vi "DIO_Configure.vi"(7 "Device Index":i32 format="%.0g", 8 "error in (no error)":errorcluster, 9 "OutBytes":T1 {"Out Byte 3" format="%08b"; "Out Byte 2" format="%08b"; "Out Byte 1" format="%08b"; "Out Byte 0" format="%08b"}, 10 "Out Mask":T2, 11 "Tri State":enum8{"False", "True"}(ring)) -> (0 "error out":errorcluster)   [LabVIEW 2012]
doc: "This VI is used to configure ACCES USB-DIO devices."
uses:
  Controls/DIO_bitMask.ctl
  Controls/DIO_bytemask.ctl
  Windows/System32/AIOUSB.dll
panel:
  out "Return Value":u32 format="%.0g"
  # "Output Bytes"
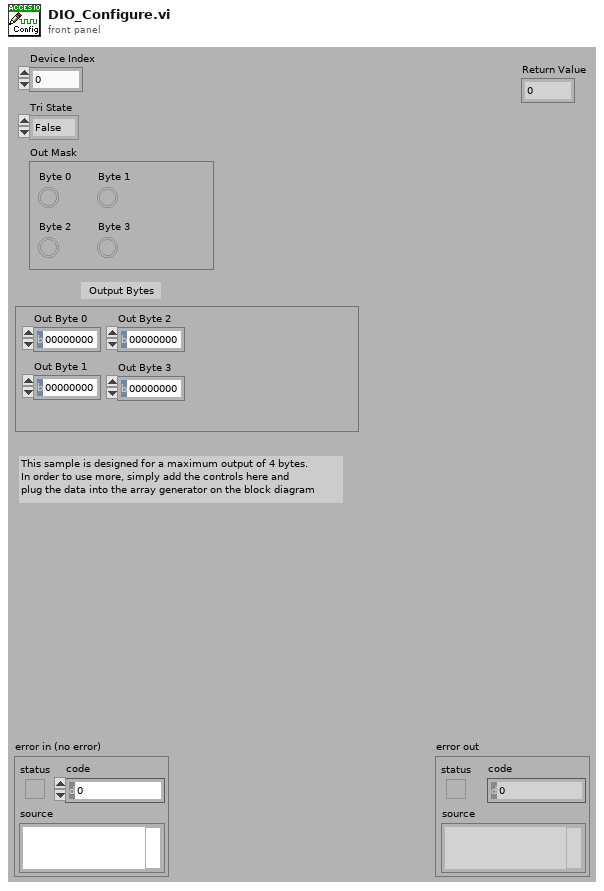
[diagram p1: front panel]
types:
  T1 = typedef "DIO_bytemask.ctl" = cluster{"Out Byte 0":u8, "Out Byte 1":u8, "Out Byte 2":u8, "Out Byte 3":u8}
  T2 = typedef "DIO_bitMask.ctl" = cluster{"Byte 0":bool, "Byte 1":bool, "Byte 2":bool, "Byte 3":bool}
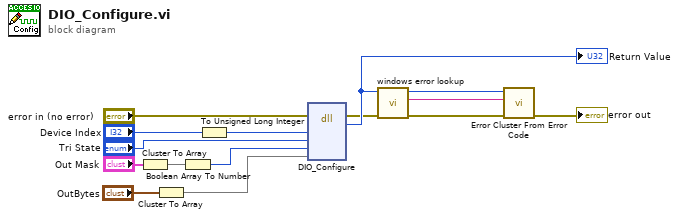
[diagram p0: block diagram]
diagram:
  n1 = Cluster To Array(cluster="Out Mask") -> (array=w3:bool[])
  n2 = Cluster To Array(cluster="OutBytes") -> (array=w5:u8[])
  n3 = Boolean Array To Number(Boolean array=w3) -> (number=w2:u32)
  n4 = To Unsigned Long Integer(number="Device Index") -> (unsigned 32bit integer=w1:u32)
  n5 = dll-call lib="C:/Windows/System32/AIOUSB.dll" fn="DIO_Configure"(error in="error in (no error)", "DeviceIndex"=w1, "bTristate"="Tri State", "pOutMask"=w2, "pData"=w5) -> (error out=w8:errorcluster, "return type"=w9:u32)  [unwired: 6 in, 1 out]
  "Return Value" <- w9
  n6 = call "windows error lookup.vi"("error in (no error)"=w8, "Error Code"=w9) -> ("error out"=w10:errorcluster, "error message (\"\")"=w11:string)  [unwired: 8 in]
  n7 = call <vilib>:"Error Cluster From Error Code.vi"("error in (no error)"=w10, "error message (\"\")"=w11, "error code (0)"=w9) -> ("error out"=→"error out":errorcluster)  [unwired: 6 in]
